vi "LoadLatestModuleInVisualizationSubPanel.vi"(8 "Error Array In in":errorcluster[](array[cluster])) -> (0 "Error Array In out":errorcluster[](array[cluster]))   [LabVIEW 2018]
uses:
  VisualizationManagerActions.ctl
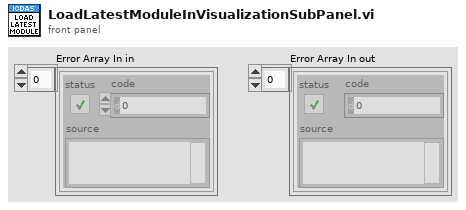
[diagram p1: front panel]
types:
  T1 = typedef "cntlRefs.ctl" = cluster{"rngFGen":refnum<vi>, "rngDigitizer":refnum<vi>, "btnHide":refnum<vi>, "rngInst":refnum<vi>, "Instrument Modules":refnum<vi>, "RelativePathToINIFiles ":refnum<vi>, "PluginTree":refnum<vi>, "TestListboxRef":refnum<vi>, "path.tstFile":refnum<vi>, "cmbxRunningModules":refnum<vi>, "TestDataSubPanel":refnum<vi>, "TestDataCaption":refnum<vi>, "btnPopInOut":refnum<vi>, "PluginMgrQ":refnum<queue>, "TestMgrQ":refnum<queue>, "TestMgrSubPanel":refnum<vi>, "PluginMgrSubPanel":refnum<vi>, "PwrReqHandle":u32, "btnStopOneTest":refnum<vi>, "pathUserfiles":refnum<vi>, "PluginTreeCaption":refnum<vi>, "MainVIRef":refnum<vi>, "btnStatus":refnum<vi>}
  T2 = typedef "VisualizationManagerActions.ctl" = enum16{"Set", "LoadModVI", "PopInOutModVI", "Add", "Clear", "CloseVisMod", "LoadLatestModule", "Get"}
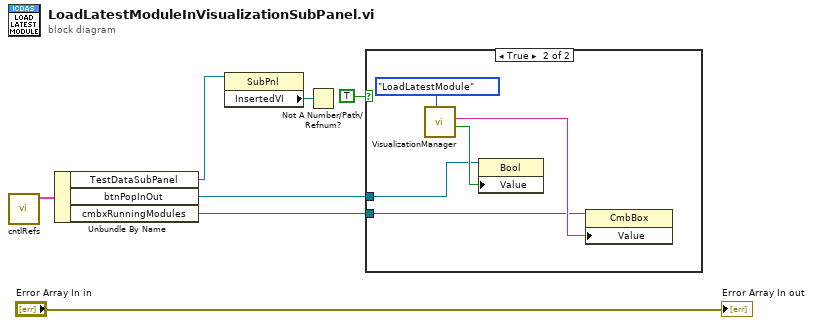
[diagram p0: block diagram]
diagram:
  n1 = call "cntlRefs.vi"() -> ("cntlRefs"=w4:T1)  [unwired: 10 in, 1 out]
  n2 = Unbundle By Name(w4) -> ("TestDataSubPanel"=w3:refnum<vi>, "btnPopInOut"=w7:refnum<vi>, "cmbxRunningModules"=w5:refnum<vi>)
  n3 = property class="SubPnl"(reference=w3) -> ("InsertedVI"=w2:refnum<vi>)  [unwired: 1 in, 2 out]
  n4 = Not A Number/Path/Refnum?(number/path/refnum=w2) -> ()  [unwired: 1 out]
  n5 = case shown="True" TRUE {
    tunnel: w7 -> [_ w11]
    tunnel: w5 -> [_ w9]
    frame False {
    }
    frame True {
      n6 = call "VisualizationManager.vi"("Action"=VisualizationManagerActions."LoadLatestModule") -> ("In SubPanel?"=w12:bool, "Module Name out"=w10:string)  [unwired: 7 in, 2 out]
      n7 = property class="Bool"(reference=w11, "Value"=w12) -> ()  [unwired: 1 in, 2 out]
      n8 = property class="CmbBox"(reference=w9, "Value"=w10) -> ()  [unwired: 1 in, 2 out]
    }
  }
  "Error Array In out" <- "Error Array In in"
